vi "Read New Mentions - Continuous.vi"() -> ()   [LabVIEW 2011]
doc: "This example gets new mentions that were posted continuously.\n\nThis example can be used to monitor for @mentions of the authenticated user."
uses:
  Controls/Tweet.ctl
  SubVIs/Twitter Open - Desktop.vi
  Mentions/Get Mentions New.vi
  i3-twitter.lvlib
panel:
  out "Mentions Read":T1[](array[typedef])
  in  "stop":bool
  out "Time Stamp of Newest Mentions":timestamp
  out "Num of Mentions Read":i32
  in  "Num of Mentions to Read":i32=10
  in  "Consumer Key":string
  in  "Consumer Secret":string
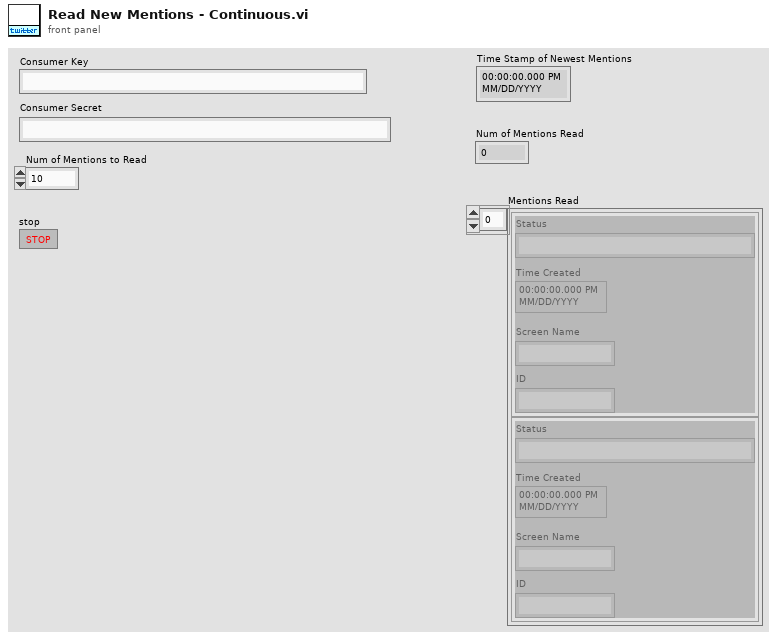
[diagram p1: front panel]
types:
  T1 = typedef "i3-twitter.lvlib/Tweet.ctl" = cluster{"Status":string, "Time Created":timestamp, "Screen Name":string, "ID":string}
  T2 = typedef "i3-oauth.lvlib/Credentials.ctl" = cluster{"Token":string, "Secret":string}
  T3 = typedef "i3-twitter.lvlib/Twitter Handle.ctl" = cluster{"OAuth Credentials":T4, "since ID":string, "max ID":string, "Screen Name":string}
  T4 = typedef "i3-oauth.lvlib/OAuth Handle.ctl" = cluster{"Signature Method":T5, "Version":string, "Client":T2, "Access":T2}
  T5 = typedef "i3-oauth.lvlib/Signature Method.ctl" = enum16{"HMAC-MD5", "HMAC-SHA1", "HMAC-SHA224", "HMAC-SHA256", "HMAC-SHA384", "HMAC-SHA512"}
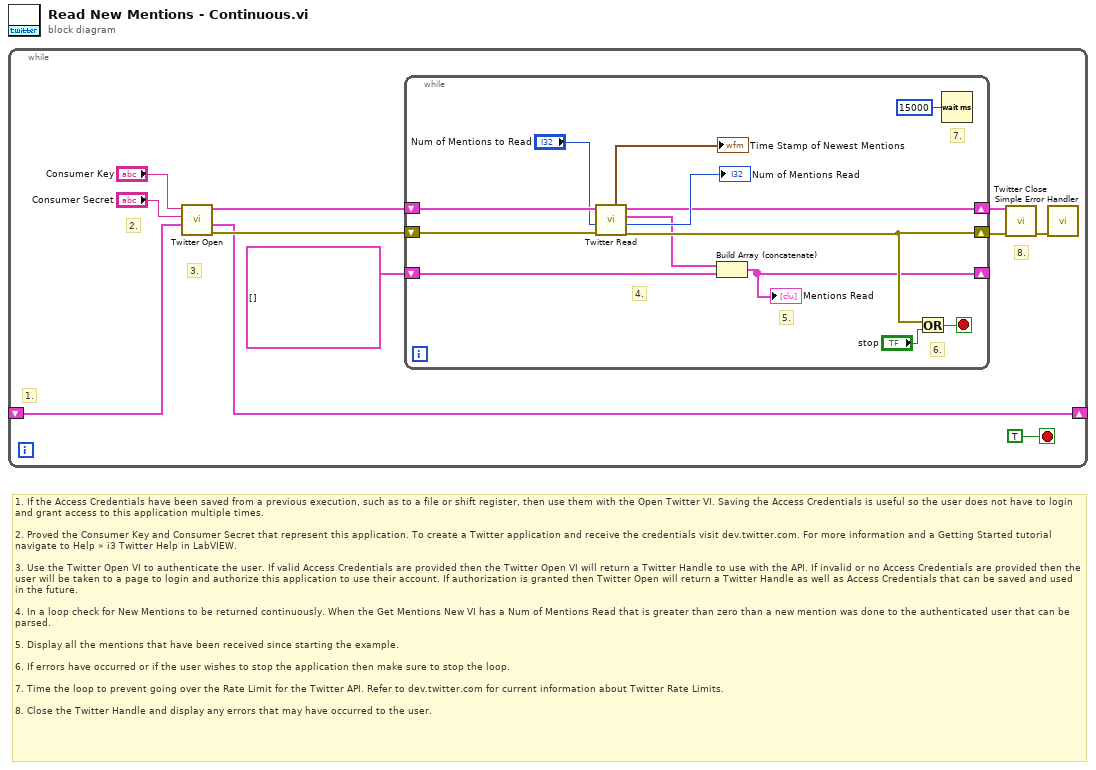
[diagram p0: block diagram]
diagram:
  # "1. If the Access Credentials have been saved from a previous execution, such as to a file or shift register, then use them with the Open Twitter VI. Saving the Access Credentials is useful so the user does not have to login and grant access to this application multiple times.\n\n2. Proved the Consumer Key and Consumer Secret that represent this application. To create a Twitter application and receive the credentials visit dev.twitter.com. For more information and a Getting Started tutorial navigate to Help » i3 Twitter Help in LabVIEW.\n\n3. Use the Twitter Open VI to authenticate the user. If valid Access Credentials are provided then the Twitter Open VI will return a Twitter Handle to use with the API. If invalid or no Access Credentials are provided then the user will be taken to a page to login and authorize this application to use their account. If authorization is granted then Twitter Open will return a Twitter Handle as well as Access Credentials that can be saved and used in the future.\n\n4. In a loop check for New Mentions to be returned continuously. When the Get Mentions New VI has a Num of Mentions Read that is greater than zero than a new mention was done to the authenticated user that can be parsed.\n\n5. Display all the mentions that have been received since starting the example.\n\n6. If errors have occurred or if the user wishes to stop the application then make sure to stop the loop.\n\n7. Time the loop to prevent going over the Rate Limit for the Twitter API. Refer to dev.twitter.com for current information about Twitter Rate Limits.\n\n8. Close the Twitter Handle and display any errors that may have occurred to the user."
  n1 = while {
    shift-right: [w2] -> _
    shift-left: _ -> [w1]
    stop <- TRUE stop-if-true
    # "1."
    # "8."
    # "3."
    # "2."
    n2 = call-poly "Twitter Open.vi"("Access Credentials (in)"=w1, "Consumer Secret"="Consumer Secret", "Consumer Key"="Consumer Key") -> ("error out"=w5:errorcluster, "Access Credentials (out)"=w2:T2, "Twitter Handle Out"=w9:T3)  [unwired: 6 in]
    n3 = while {
      shift-right: [w20] -> w7
      shift-left: w9 -> [w22]
      shift-right: [w18] -> _
      shift-left: T1[] [] ("Tweets Array") -> [w13]
      shift-right: [w23] -> w8
      shift-left: w5 -> [w21]
      stop <- w16 stop-if-true
      # "7."
      # "6."
      # "5."
      # "4."
      n4 = call-poly "Twitter Read.vi"("error in"=w21, "Mentions to Read (10)"="Num of Mentions to Read", "Twitter Handle In"=w22) -> ("error out"=w23:errorcluster, "Actual Num of Mentions Read"=→"Num of Mentions Read":i32, "New Mentions Read"=w14:T1[], "Twitter Handle Out"=w20:T3, "Time Stamp of Newest Mention"=→"Time Stamp of Newest Mentions":timestamp)  [unwired: 4 in]
      n5 = Build Array (concatenate)(w14, w13) -> (w18:T1[])
      "Mentions Read" <- w18
      n6 = Or(x=w23, y="stop") -> (x .or. y?=w16:bool)
      n7 = Wait (ms)(milliseconds to wait=u32 15000) -> ()  [unwired: 1 out]
    }
    n8 = call "Twitter Close.vi"("error in"=w8, "Twitter Handle In"=w7) -> ("error out"=w3:errorcluster)  [unwired: 9 in]
    n9 = call <vilib>:"Simple Error Handler.vi"("error in (no error)"=w3) -> ()  [unwired: 4 in, 5 out]
  }
